vi "Remove Empty Array.vi"   [LabVIEW 2020]
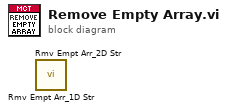
[diagram p0: block diagram]
diagram:
  n1 = call "Rmv Empt Arr_1D Str.vi"() -> ()  [unwired: 10 in, 2 out]
  n2 = call "Rmv Empt Arr_2D Str.vi"() -> ()  [unwired: 10 in, 2 out]
